vi "Occupied Resources.vi"(7 "Rate Class":T1, 8 "error in":errorcluster, 10 "Chassis Name":string, 11 "Chassis Cfg":refnum<class "ChassisCfg.lvclass">) -> (0 "error out":errorcluster, 2 "Taken Dual Rate Mods":string[](array[string]), 3 "All Chassis/Chan Names":string[](array[string]))   [LabVIEW 2018, in "Configuration Grandmaster.lvlib" / "ChassisCfg.lvclass"]
uses:
  ChassisCfg.lvclass
  Common/Controls/TE_Designator.ctl
  ChassisCfg.lvclass/ChassisCfg.ctl
  Class Timing Group/TimingGrp.lvclass
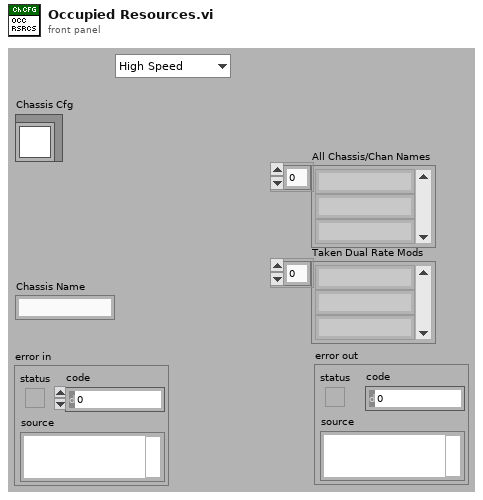
[diagram p1: front panel]
types:
  T1 = typedef "TE_Designator.ctl" = enum16{"High Speed", "Low Speed"}
  T2 = typedef "ge_MultiRateMods.ctl" = cluster{"NI 9205":bool, "NI 9221":bool}
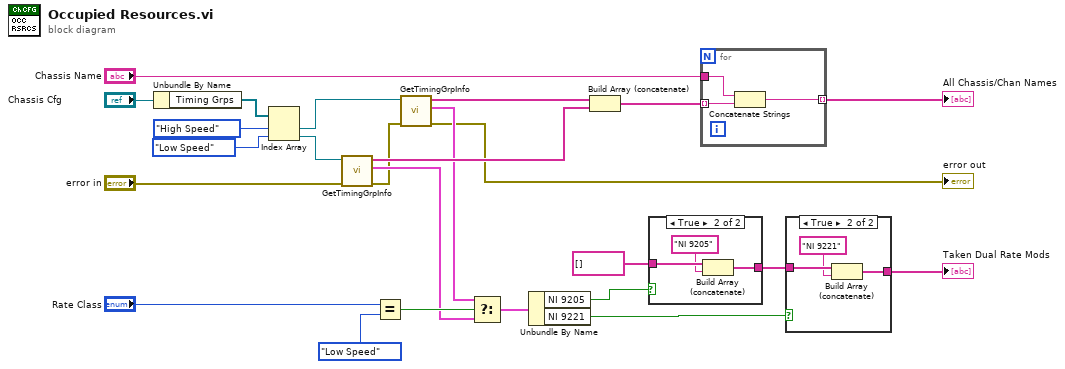
[diagram p0: block diagram]
diagram:
  n1 = Unbundle By Name("Chassis Cfg") -> ("Timing Grps"=w3:refnum<class "TimingGrp.lvclass">[])
  n2 = Index Array(array=w3, index #1=TE_Designator."High Speed" ("Timing Engine"), index #2=TE_Designator."Low Speed" ("Timing Engine")) -> (element #1=w2:refnum<class "TimingGrp.lvclass">, element #2=w1:refnum<class "TimingGrp.lvclass">)
  n3 = call "GetTimingGrpInfo.vi"("error in"="error in", "TimingGrp in"=w1) -> ("error out"=w11:errorcluster, "Multi Rate Mods in Timing Grp"=w16:T2, "All TimingGrp Chans"=w21:string[])  [unwired: 4 in, 3 out]
  n4 = Equal?(x="Rate Class", y=TE_Designator."Low Speed") -> (x = y?=w18:bool)
  n5 = call "GetTimingGrpInfo.vi"("error in"=w11, "TimingGrp in"=w2) -> ("error out"=→"error out":errorcluster, "Multi Rate Mods in Timing Grp"=w17:T2, "All TimingGrp Chans"=w25:string[])  [unwired: 4 in, 3 out]
  n6 = Select(t=w17, s=w18, f=w16) -> (s? t:f=w15:T2)
  n7 = Unbundle By Name(w15) -> ("NI 9205"=w14:bool, "NI 9221"=w13:bool)
  n8 = Build Array (concatenate)(w25, w21) -> (w8:string[])
  n9 = case shown="True" w14 {
    tunnel: string[] [] -> [w26 w29]
    tunnel: [w26 w27] -> w22
    frame False {
    }
    frame True {
      n10 = Build Array (concatenate)(w29, "NI 9205") -> (w27:string[])
    }
  }
  n11 = for {
    tunnel: w8 -> [w31] mode=indexing
    tunnel: "Chassis Name" -> [w32]
    tunnel: [w30] -> w6 mode=indexing
    n12 = Concatenate Strings(w32, w31) -> (w30:string)
  }
  "All Chassis/Chan Names" <- w6
  n13 = case shown="True" w13 {
    tunnel: w22 -> [w33 w36]
    tunnel: [w33 w34] -> w12
    frame False {
    }
    frame True {
      n14 = Build Array (concatenate)(w36, "NI 9221") -> (w34:string[])
    }
  }
  "Taken Dual Rate Mods" <- w12
